vi "Error-Get All Errors From List.vi"(0 "Path":path) -> (4 "Codes":i32[](array[numeric]), 6 "Errors":T1[](array[typedef]), 15 "error out":errorcluster)   [LabVIEW 2020]
uses:
  Error Description.ctl
  <vilib>/regexp/Match Regular Expression.xnode
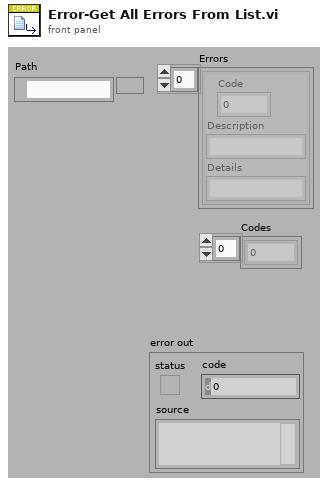
[diagram p1: front panel]
types:
  T1 = typedef "Error Description.ctl" = cluster{"Code":i32, "Description":string, "Details":string}
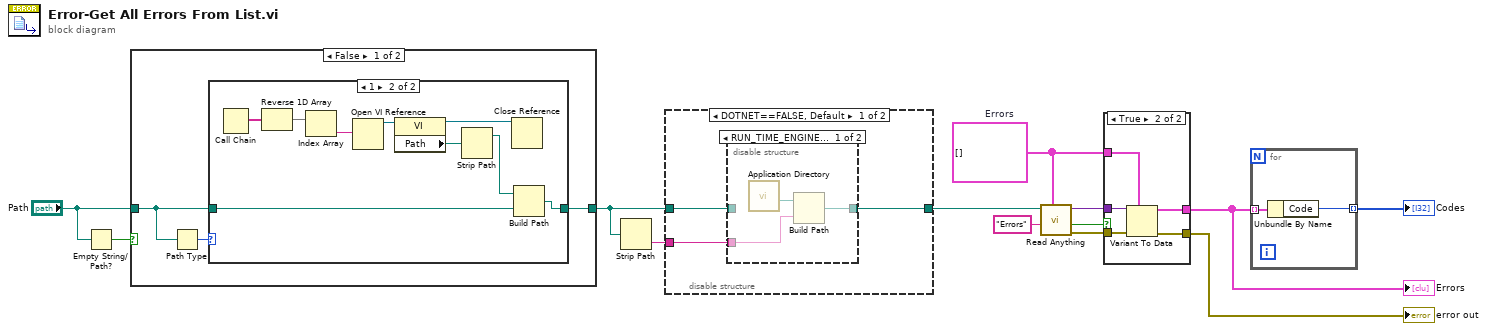
[diagram p0: block diagram]
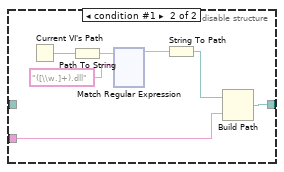
[diagram p3: hidden frame]
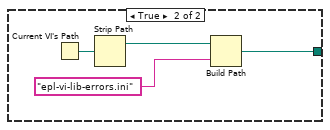
[diagram p5: hidden frame]
diagram:
  w10 = T1[] []  # Errors
  n1 = Empty String/Path?(string/path="Path") -> (empty?=w5:bool)
  n2 = case shown="False" w5 {
    tunnel: [w15 w30] -> w3
    tunnel: "Path" -> [w14 _]
    frame False {
      n3 = Path Type(1:w14) -> (0:w16:i16)
      n4 = case shown="1" w16 {
        tunnel: [w17 w25] -> w15
        tunnel: w14 -> [w17 w26]
        frame 0, Default {
        }
        frame 1 {
          n5 = Call Chain() -> (call chain=w24:string[])
          n6 = Reverse 1D Array(array=w24) -> (reversed array=w23:string[])
          n7 = Index Array(array=w23) -> (element=w22:string)  [unwired: 1 in]
          n8 = Open VI Reference(vi path=w22) -> (vi reference=w21:refnum<vi>)  [unwired: 5 in, 1 out]
          n9 = property class="VI"(reference=w21) -> (reference out=w20:refnum<vi>, "Path"=w19:path)  [unwired: 1 in, 1 out]
          n10 = Strip Path(path=w19) -> (stripped path=w18:path)  [unwired: 1 out]
          n11 = Close Reference(reference=w20) -> ()  [unwired: 1 in, 1 out]
          n12 = Build Path(base path=w18, name or relative path=w26) -> (appended path=w25:path)
        }
      }
    }
    frame True {
      n13 = Current VI's Path() -> (path=w28:path)
      n14 = Strip Path(path=w28) -> (stripped path=w29:path)  [unwired: 1 out]
      n15 = Build Path(base path=w29, name or relative path="epl-vi-lib-errors.ini") -> (appended path=w30:path)
    }
  }
  n16 = Strip Path(path=w3) -> (name=w2:string)  [unwired: 1 out]
  n17 = disable-structure shown="DOTNET==FALSE, Default" {
    disable-tunnel: w3 -> [w31 _]
    disable-tunnel: w2 -> [w33 w38]
    disable-tunnel: [w32 w39] -> w1
    frame condition #0 (active) {
      n18 = disable-structure shown="RUN_TIME_ENGINE==True" {
        disable-tunnel: w33 -> [w35 _]
        disable-tunnel: [w36 w37] -> w32
        disable-tunnel: w31 -> [_ w37]
        frame condition #0 {
          n19 = call <vilib>:"Application Directory.vi"() -> ("Application Directory"=w34:path)
          n20 = Build Path(base path=w34, name or relative path=w35) -> (appended path=w36:path)
        }
        frame condition #1 (active) {
        }
      }
    }
    frame condition #1 {
      n21 = Current VI's Path() -> (path=w44:path)
      n22 = Path To String(path=w44) -> (string=w43:string)
      n23 = xnode "Match Regular Expression"("input string"=w43, "regular expression"="([\\w.]+).dll") -> ("before match"=w41:string)  [unwired: 4 in, 4 out]
      n24 = String To Path(string=w41) -> (path=w40:path)
      n25 = Build Path(base path=w40, name or relative path=w38) -> (appended path=w39:path)
    }
  }
  n26 = call "Read Anything.vi"("Type of Anything"=w10, "Section Name (Name of \"Type of Anything\")"="Errors" ("Section Name (Name of \"Type of Anything\")"), "Path (dialog)"=w1) -> ("Error Out"=w7:errorcluster, "Found?"=w12:bool, "Anything"=w11:variant)  [unwired: 6 in]
  n27 = case shown="True" w12 {
    tunnel: w11 -> [_ w164]
    tunnel: w10 -> [_ w163]
    tunnel: [_ w162] -> w8
    tunnel: w7 -> [w159 w161]
    tunnel: [w159 w160] -> w6
    frame False {
    }
    frame True {
      n28 = Variant To Data(error in=w161, type=w163, Variant=w164) -> (data=w162:T1[], error out=w160:errorcluster)
    }
  }
  "error out" <- w6
  "Errors" <- w8
  n29 = for {
    tunnel: w8 -> [w166] mode=indexing
    tunnel: [w165] -> w13 mode=indexing
    n30 = Unbundle By Name(w166) -> ("Code"=w165:i32)
  }
  "Codes" <- w13
